vi "Write Pct Encode.vi"(8 "error in (no error)":errorcluster, 10 "Pct Encode":bool, 11 "URI-Component in":refnum<class "URI-Component.lvclass">) -> (0 "error out":errorcluster, 3 "URI-Component out":refnum<class "URI-Component.lvclass">)   [LabVIEW 2013, in "openURI.lvlib" / "URI-Component.lvclass"]
uses:
  URI-Component.lvclass
  URI-Component.lvclass/URI-Component.ctl
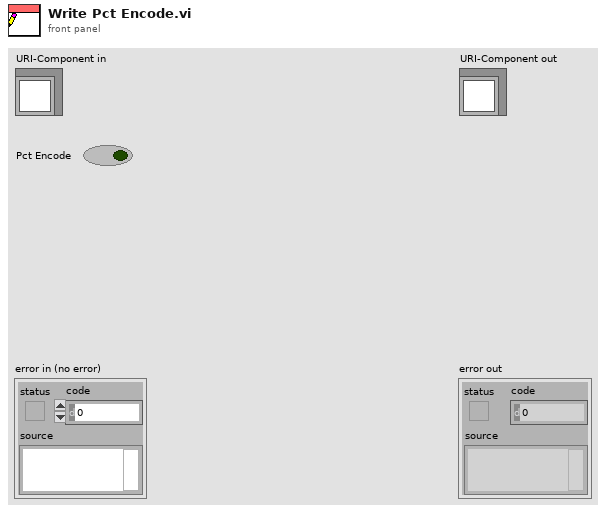
[diagram p1: front panel]
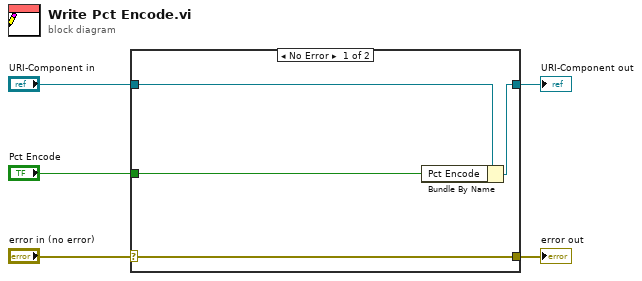
[diagram p0: block diagram]
diagram:
  n1 = case shown="No Error" "error in (no error)" {
    selector: "error in (no error)" -> [w9 w10]
    tunnel: [w9 w10] -> w4
    tunnel: [w7 w11] -> w2
    tunnel: "URI-Component in" -> [w8 w11]
    tunnel: "Pct Encode" -> [w6 _]
    frame No Error {
      n2 = Bundle By Name(cluster=w8, "Pct Encode"=w6) -> (w7:refnum<class "URI-Component.lvclass">)
    }
    frame Error {
    }
  }
  "error out" <- w4
  "URI-Component out" <- w2
